vi "WriteCmd.vi"(4 "error in (no error)":errorcluster, 6 "write buffer":string, 7 "VISA Refnum in":refnum<visa-resource-name>) -> (0 "error out":errorcluster, 2 "Valid":bool, 3 "VISA Refnum out":refnum<visa-resource-name>)   [LabVIEW 2015, in "Ion Motion Roboclaw.lvlib"]
uses:
  <instrlib>/Ion Motion Roboclaw/Ion Motion Roboclaw.lvlib
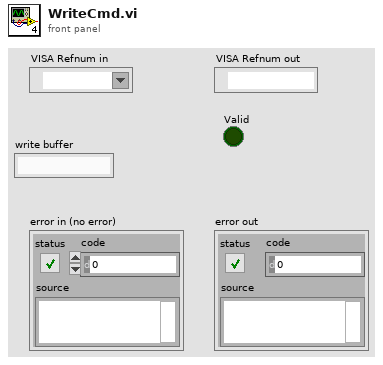
[diagram p1: front panel]
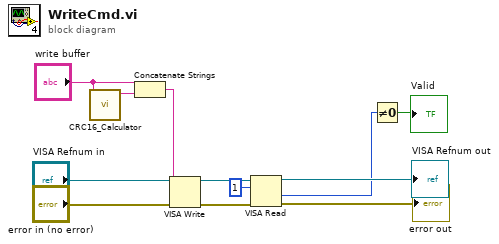
[diagram p0: block diagram]
diagram:
  n1 = call <instrlib>:"CRC16_Calculator.vi"("String in"="write buffer") -> ("CRC16 out"=w4:string)  [unwired: 8 in, 2 out]
  n2 = Concatenate Strings("write buffer", w4) -> (w1:string)
  n3 = VISA Write(VISA resource name="VISA Refnum in", write buffer=w1, error in (no error)="error in (no error)") -> (VISA resource name out=w12:refnum<visa-resource-name>, error out=w11:errorcluster)  [unwired: 1 out]
  n4 = VISA Read(VISA resource name=w12, byte count=u32 1, error in (no error)=w11) -> (VISA resource name out=→"VISA Refnum out":refnum<visa-resource-name>, return count=w7:u32, error out=→"error out":errorcluster)  [unwired: 1 out]
  n5 = Not Equal To 0?(x=w7) -> (x != 0?=→"Valid":bool)
